vi "Example Graph.vi"() -> ()   [LabVIEW 2013]
uses:
  C:/tf/play/labview/Tinkerforge.dll
  Tinkerforge.dll
panel:
  in  "stop":bool
  out "graph":sgl[](graph)
  in  "uid":string="amb"
  in  "port":i32=4223
  in  "host":string="localhost"
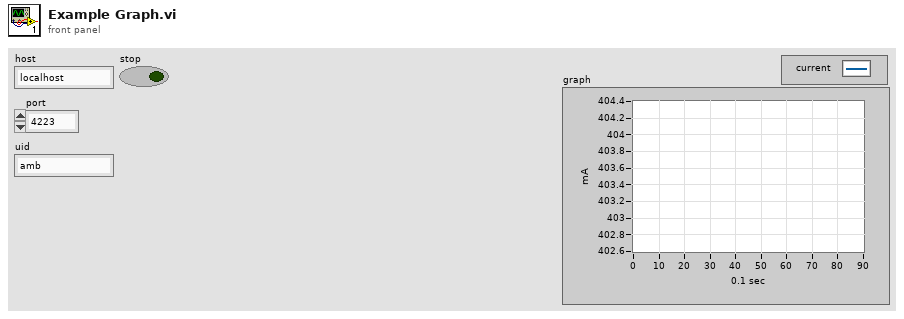
[diagram p1: front panel]
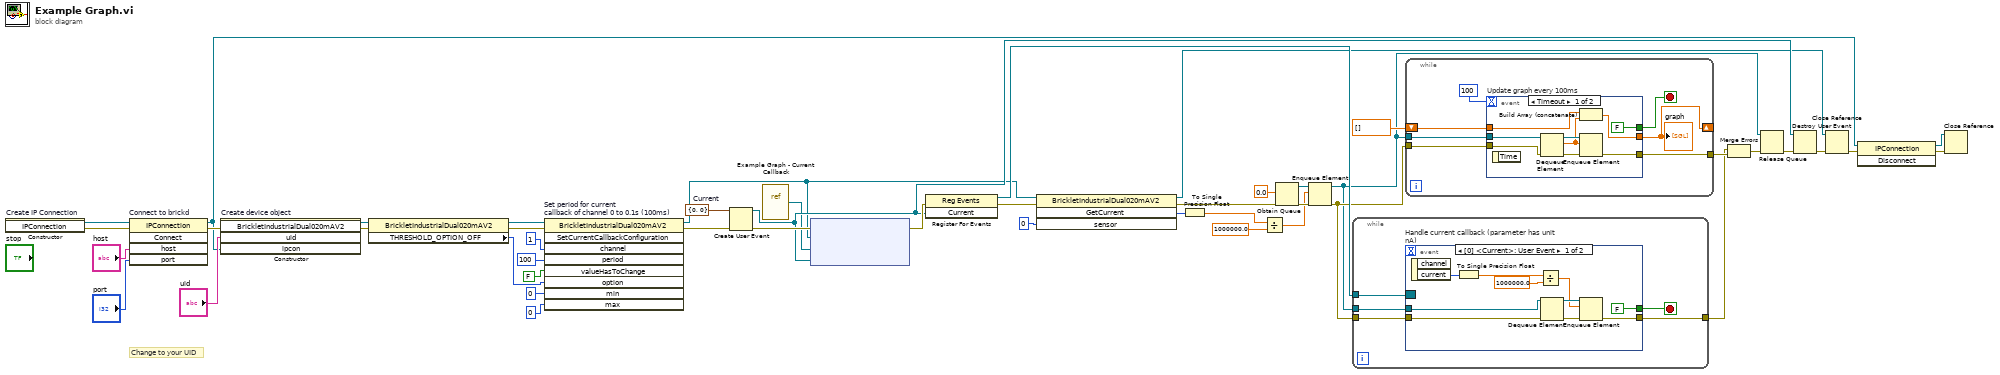
[diagram p0: block diagram]
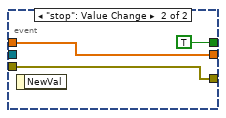
[diagram p2: hidden frame]
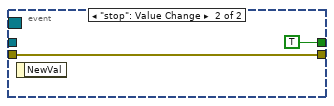
[diagram p3: hidden frame]
diagram:
  w33 = cluster{"channel":u8, "current":i32} {"channel"=0, "current"=0}  # Current
  # "Change to your UID"
  n1 = constructor on="Create IP Connection" class="IPConnection"() -> (reference out=w47:refnum<k24>, error out=w20:errorcluster)  [unwired: 3 in, 1 out]
  n2 = invoke on="Connect to brickd" class="IPConnection" method="Connect"(reference=w47, error in=w20, "host"="host", "port"="port") -> (reference out=w40:refnum<k24>, error out=w43:errorcluster)  [unwired: 1 in, 3 out]
  n3 = constructor on="Create device object" class="BrickletIndustrialDual020mAV2"(error in=w43, "uid"="uid", "ipcon"=w40) -> (reference out=w9:refnum<k24>, error out=w6:errorcluster)  [unwired: 2 in, 3 out]
  n4 = property class="BrickletIndustrialDual020mAV2"(reference=w9, error in=w6) -> (reference out=w8:refnum<k24>, error out=w7:errorcluster, "THRESHOLD_OPTION_OFF"=w4:u16)
  n5 = invoke on="Set period for current\ncallback of channel 0 to 0.1s (100ms)" class="BrickletIndustrialDual020mAV2" method="SetCurrentCallbackConfiguration"(reference=w8, error in=w7, "channel"=u8 1 ("sensor"), "period"=i64 100, "valueHasToChange"=FALSE, "option"=w4, "min"=0, "max"=0) -> (reference out=w17:refnum<k24>, error out=w32:errorcluster)  [unwired: 1 in, 7 out]
  n6 = Create User Event(user event datatype=w33, error in=w32) -> (user event=w35:refnum<user-event>, error out=w38:errorcluster)
  n7 = vi-ref "Example Graph - Current Callback.vi"() -> ("vi reference"=w1:refnum<vi>)
  n8 = node ("Register Event Callback")(w38, w17, w1, w35) -> (w37:errorcluster)  [unwired: 1 in, 1 out]
  n9 = register-events(error in=w37, w35) -> (reference out=w36:refnum<event-registration>, error out=w19:errorcluster)  [unwired: 1 in]
  n10 = invoke class="BrickletIndustrialDual020mAV2" method="GetCurrent"(reference=w17, error in=w19, "sensor"=u8 0) -> (reference out=w16:refnum<k24>, error out=w18:errorcluster, "GetCurrent"=w13:i32)  [unwired: 1 in, 1 out]
  n11 = To Single Precision Float(number=w13) -> (single precision float=w15:sgl)
  n12 = Divide(x=w15, y=sgl 1000000.0) -> (x/y=w12:sgl)
  n13 = Obtain Queue(element data type=sgl 0.0, error in (no error)=w18) -> (queue out=w24:refnum<queue>, error out=w26:errorcluster)  [unwired: 3 in, 1 out]
  n14 = Enqueue Element(queue=w24, element=w12, error in (no error)=w26) -> (queue out=w21:refnum<queue>, error out=w25:errorcluster)  [unwired: 1 in, 1 out]
  n15 = while {
    tunnel: w36 -> [w52]
    tunnel: [w50] -> w29
    tunnel: w25 -> [w51]
    tunnel: w21 -> [w49]
    stop <- w48 stop-if-true
    n16 = event "Handle current callback (parameter has unit nA)" shown="[0] <Current>: User Event" {
      selector: w52 -> [_ _]
      dyn-events: _ -> [_ _]
      timeout: _ -> [_ _]
      tunnel: w51 -> [w60 w63]
      tunnel: [w58 w63] -> w50
      tunnel: w49 -> [w57 _]
      tunnel: [FALSE TRUE] -> w48
      event User Event {
        n17 = event-data() -> ("current"=w53:i32)  [unwired: 1 in, 1 out]
        n18 = To Single Precision Float(number=w53) -> (single precision float=w61:sgl)
        n19 = Divide(x=w61, y=sgl 1000000.0) -> (x/y=w55:sgl)
        n20 = Dequeue Element(queue=w57, error in (no error)=w60) -> (queue out=w56:refnum<queue>, error out=w59:errorcluster)  [unwired: 1 in, 2 out]
        n21 = Enqueue Element(queue=w56, element=w55, error in (no error)=w59) -> (error out=w58:errorcluster)  [unwired: 1 in, 2 out]
      }
      event "stop": Value Change {
        n22 = event-data() -> ()  [unwired: 1 in, 1 out]
      }
    }
  }
  n23 = while {
    tunnel: [w67] -> w30
    tunnel: w25 -> [w68]
    shift-right: [w69] -> _
    shift-left: sgl[] [] -> [w70]
    tunnel: w21 -> [w66]
    stop <- w65 stop-if-true
    n24 = event "Update graph every 100ms" shown="[0] Timeout" {
      selector: _ -> [_ _]
      dyn-events: _ -> [_ _]
      timeout: 100 -> [_ _]
      tunnel: [w80 w82] -> w69
      tunnel: w70 -> [w73 w82]
      tunnel: w68 -> [w79 w81]
      tunnel: [w76 w81] -> w67
      tunnel: w66 -> [w78 _]
      tunnel: [FALSE TRUE] -> w65
      event Timeout {
        n25 = event-data() -> ()  [unwired: 1 in, 1 out]
        n26 = Dequeue Element(queue=w78, error in (no error)=w79) -> (queue out=w75:refnum<queue>, element=w74:sgl, error out=w77:errorcluster)  [unwired: 1 in, 1 out]
        n27 = Build Array (concatenate)(w73, w74) -> (w80:sgl[])
        n28 = Enqueue Element(queue=w75, element=w74, error in (no error)=w77) -> (error out=w76:errorcluster)  [unwired: 1 in, 2 out]
      }
      event "stop": Value Change {
        n29 = event-data() -> ()  [unwired: 1 in, 1 out]
      }
    }
    "graph" <- w69
  }
  n30 = Merge Errors(w29, w30) -> (w23:errorcluster)
  n31 = Release Queue(queue=w21, error in (no error)=w23) -> (error out=w22:errorcluster)  [unwired: 1 in, 2 out]
  n32 = Destroy User Event(user event=w35, error in=w22) -> (error out=w34:errorcluster)
  n33 = Close Reference(reference=w16, error in (no error)=w34) -> (error out=w42:errorcluster)
  n34 = invoke class="IPConnection" method="Disconnect"(reference=w40, error in=w42) -> (reference out=w39:refnum<k24>, error out=w41:errorcluster)  [unwired: 1 in, 1 out]
  n35 = Close Reference(reference=w39, error in (no error)=w41) -> ()  [unwired: 1 out]
